vi "new square.vi"(11 "Error In":errorcluster) -> ()   [LabVIEW 2019]
uses:
  <vilib>/Platform/TimedLoop/XDataNode/timing_clust.ctl
  <vilib>/Platform/TimedLoop/XDataNode/nitl_modes.ctl
  <vilib>/Platform/TimedLoop/XDataNode/wakeup.ctl
  Global.vi
  <vilib>/platform/TimedLoop/XDataNode/XDataNode.xnode
  <vilib>/Platform/TimedLoop/XDataNode/XDNodeRunTimeDep.lvlib
panel:
  out "msec Low":dbl=400.0
  out "msec High":dbl=600.0
  out "Duty Cycle":dbl
  out "Frequency":dbl
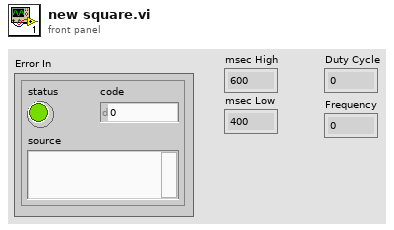
[diagram p1: front panel]
types:
  T1 = typedef "XDNodeRunTimeDep.lvlib/timing_clust.ctl" = cluster{"Expected End [f-1]":u64, "Actual End [f-1]":u64, "Finished Late? [f-1]":bool, "Expected End [i-1]":u64, "Actual End [i-1]":u64, "Finished Late? [i-1]":bool, "Expected Start [i]":u64, "Actual Start [i]":u64, "Expected Start [f]":u64, "Actual Start [f]":u64, "Source Name":string, "Structure Name":string, "Period":i64, "Deadline":i64, "Offset":i64, "Start":i64, "Priority":i32, "Timeout":i32, "Mode":T2, "Wakeup Reason":T3, "Error":errorcluster, "Source Type":string, "Secondary Source Type":string, "Global End Time":u64, "Global Start Time":u64, "Frame Duration":u64, "Iteration Duration":u64, "Assigned CPU":i32, "I/O Scan Engine Mode":u32}
  T2 = typedef "XDNodeRunTimeDep.lvlib/nitl_modes.ctl" = enum32{"No Change", "Process missed periods, maintain original phase", "Discard missed periods, maintain original phase", "Process missed periods, ignore original phase", "Discard missed periods, ignore original phase"}
  T3 = typedef "XDNodeRunTimeDep.lvlib/wakeup.ctl" = enum32{"Normal", "Aborted", "Asynchronous wakeup", "Timing source error", "Timed loop error", "Timeout"}
  T4 = cluster{"Frequency (Hz)":dbl, "Delay":dbl, "Duty cycle %":dbl}
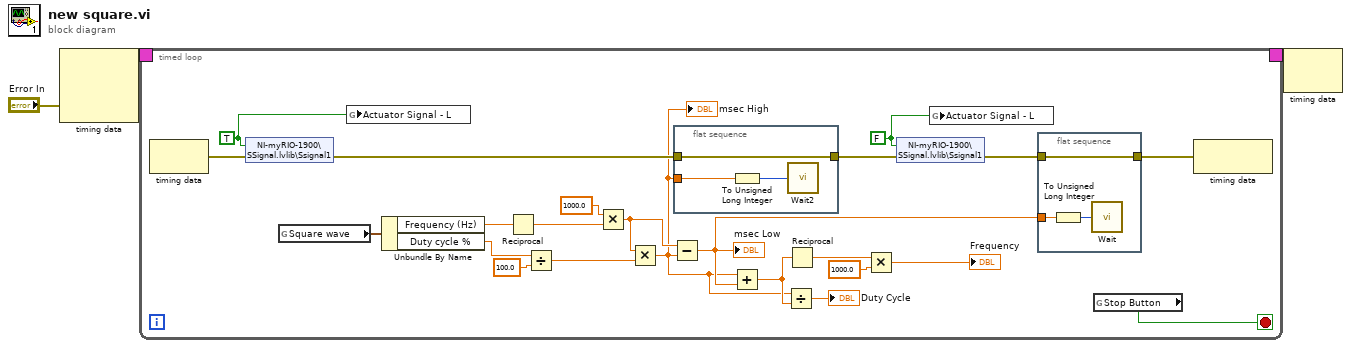
[diagram p0: block diagram]
diagram:
  n1 = node-c288("Error In") -> (w3:T1)  [unwired: 2 in]
  n2 = timed-loop {
    timing: w3 -> [_]
    timing-out: [_] -> w2
    stop <- w21 stop-if-true
    w5 = FALSE ("DO0")
    w4 = TRUE ("DO0")
    n3 = node-c288() -> (w20:errorcluster)  [unwired: 1 in]
    n4 = shared-variable "NI-myRIO-1900\\SSignal.lvlib\\Ssignal1"(w4, error in=w20) -> (error out=w25:errorcluster)
    n5 = global read "Global.vi" "Square wave"() -> (w18:T4)
    n6 = global write "Global.vi" "Actuator Signal - L"(w4) -> ()
    n7 = Unbundle By Name(w18) -> ("Frequency (Hz)"=w17:dbl, "Duty cycle %"=w14:dbl)
    n8 = Reciprocal(x=w17) -> (1/x=w16:dbl)
    n9 = Divide(x=w14, y=100.0) -> (x/y=w12:dbl)
    n10 = Multiply(x=1000.0, y=w16) -> (x*y=w13:dbl)
    n11 = Multiply(x=w13, y=w12) -> (x*y=w6:dbl)
    "msec High" <- w6
    n12 = Subtract(x=w13, y=w6) -> (x-y=w7:dbl)
    "msec Low" <- w7
    n13 = flat-sequence {
      tunnel: w6 -> [w34]
      tunnel: w25 -> [w33]
      tunnel: [w33] -> w24
      frame #0 {
        n14 = To Unsigned Long Integer(number=w34) -> (unsigned 32bit integer=w32:u32)
        n15 = call "Wait2"("Count(mSec)"=w32) -> ()  [unwired: 1 out]
      }
    }
    n16 = Add(x=w6, y=w7) -> (x+y=w22:dbl)
    n17 = Divide(x=w6, y=w22) -> (x/y=→"Duty Cycle":dbl)
    n18 = Reciprocal(x=w22) -> (1/x=w11:dbl)
    n19 = Multiply(x=w11, y=1000.0) -> (x*y=→"Frequency":dbl)
    n20 = shared-variable "NI-myRIO-1900\\SSignal.lvlib\\Ssignal1"(w5, error in=w24) -> (error out=w23:errorcluster)
    n21 = global write "Global.vi" "Actuator Signal - L"(w5) -> ()
    n22 = flat-sequence {
      tunnel: w23 -> [w37]
      tunnel: [w37] -> w19
      tunnel: w7 -> [w36]
      frame #0 {
        n23 = To Unsigned Long Integer(number=w36) -> (unsigned 32bit integer=w35:u32)
        n24 = call "Wait"("Count(mSec)"=w35) -> ()  [unwired: 1 out]
      }
    }
    n25 = global read "Global.vi" "Stop Button"() -> (w21:bool)
    n26 = node-c288(w19) -> ()  [unwired: 1 out]
  }
  n27 = node-c288(w2) -> ()  [unwired: 1 out]
